vi "BasicIO.vi"() -> ()   [LabVIEW 2020]
panel:
  out "String Indicator":string
  in  "String Control":string
  out "Boolean Switch":bool
  in  "Boolean Switch":bool
  out "Numeric Indicator":dbl
  in  "Numeric Control":dbl
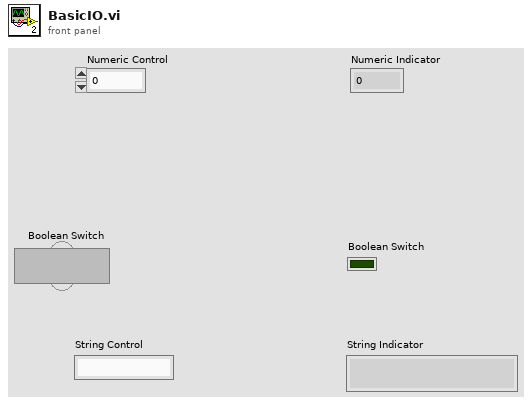
[diagram p1: front panel]
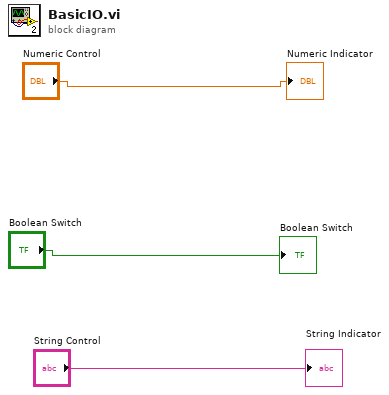
[diagram p0: block diagram]
diagram:
  "Numeric Indicator" <- "Numeric Control"
  "Boolean Switch" <- "Boolean Switch"
  "String Indicator" <- "String Control"
